vi "Heater Control.vi"(8 "error in":errorcluster, 11 "HeatFlow Results in":refnum<class "Heat Flow Results.lvclass">) -> (0 "error out":errorcluster, 1 "Ugs Cold":dbl caption="Ugs Cold, V", 2 "Ugs Hot":dbl caption="Ugs Hot, V", 3 "HeatFlow Results out":refnum<class "Heat Flow Results.lvclass">)   [LabVIEW 2019, in "Results.lvlib" / "Heat Flow Results.lvclass"]
uses:
  Heat Flow Results.lvclass
  Heat Flow Results.lvclass/Heat Flow Results.ctl
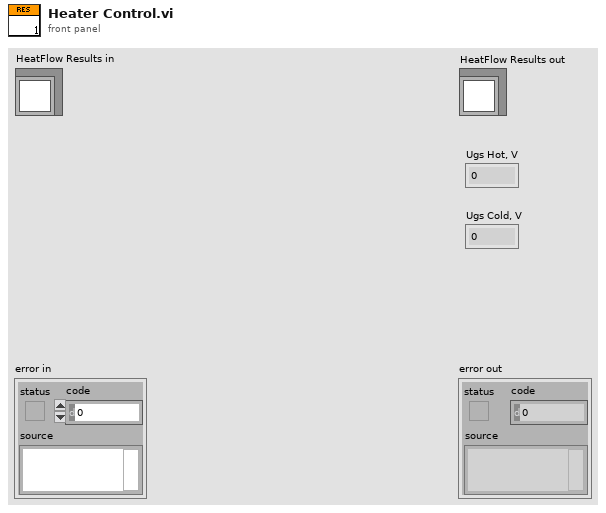
[diagram p1: front panel]
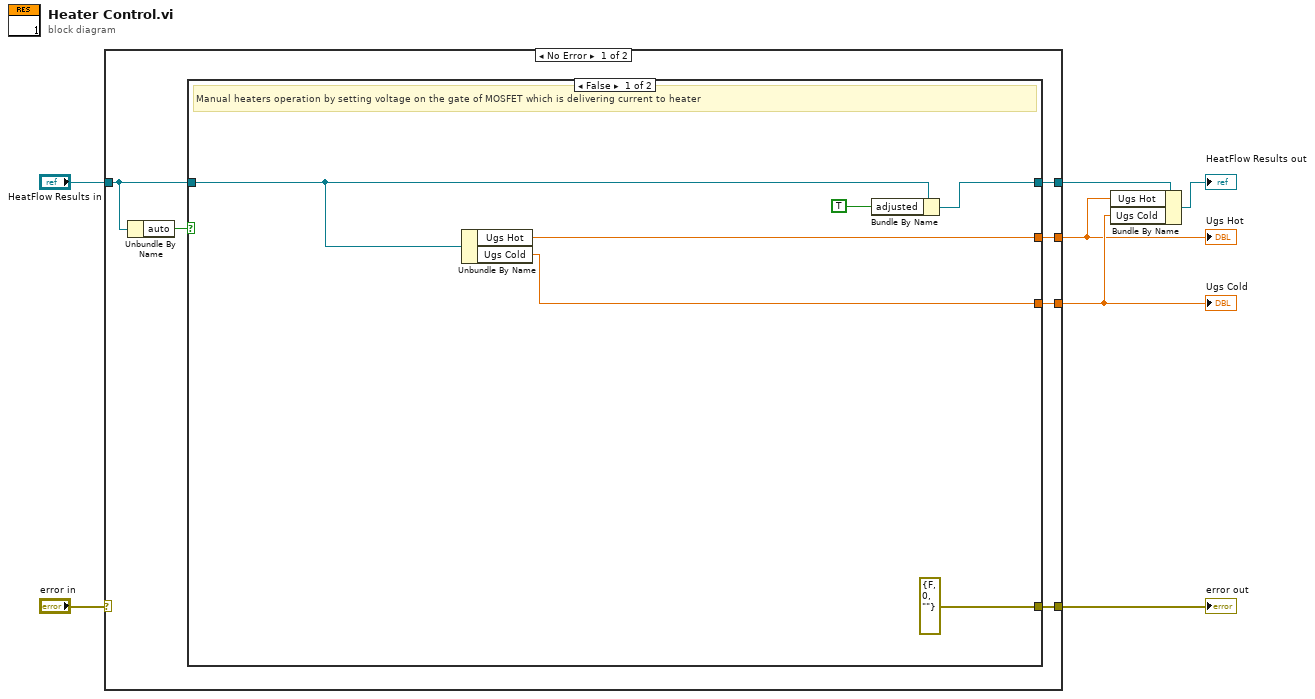
[diagram p0: block diagram]
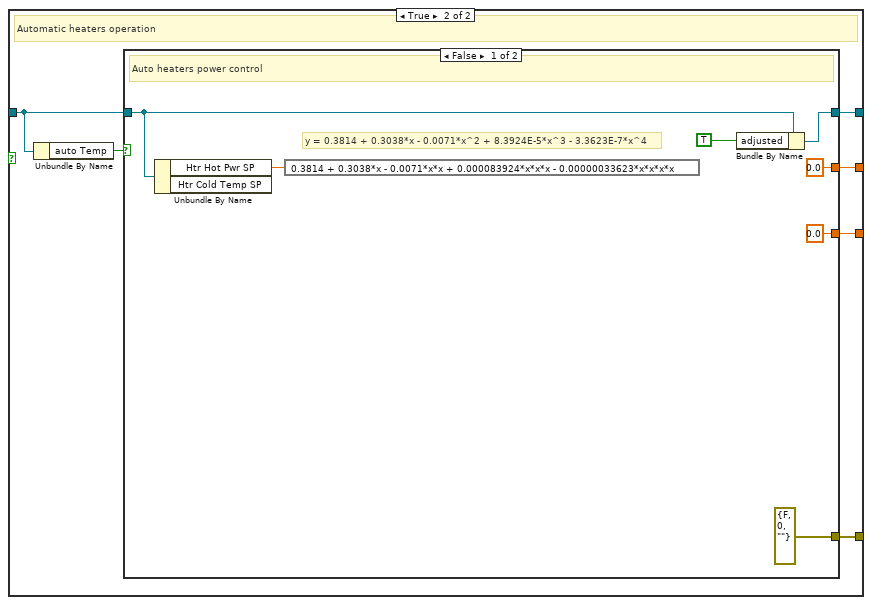
[diagram p2: hidden frame]
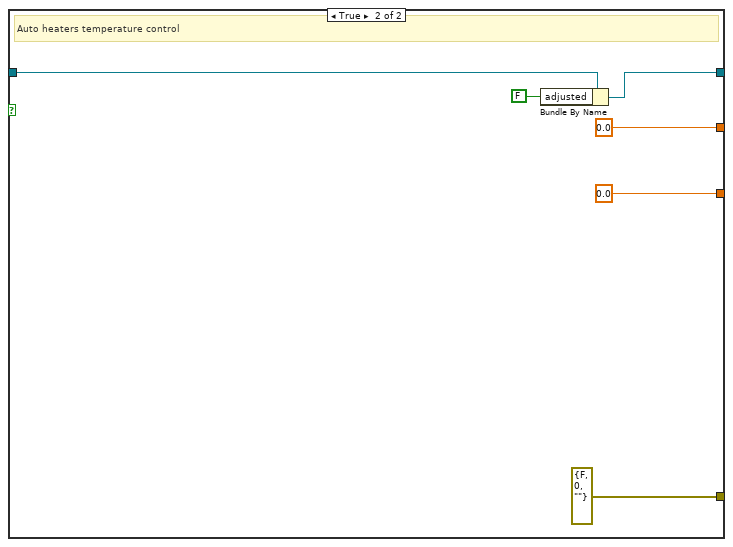
[diagram p3: hidden frame]
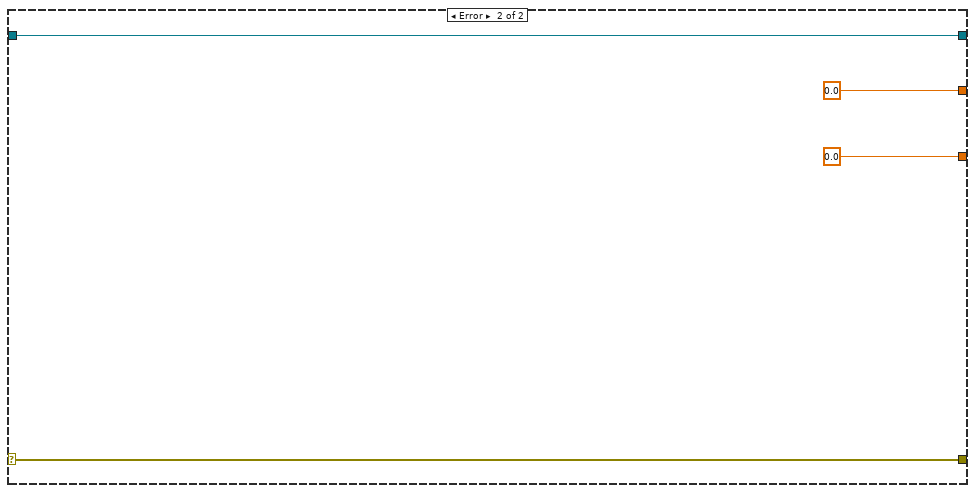
[diagram p4: hidden frame]
diagram:
  n1 = case shown="No Error" "error in" {
    selector: "error in" -> [_ w42]
    tunnel: [w10 w42] -> w6
    tunnel: "HeatFlow Results in" -> [w12 w40]
    tunnel: [w13 0.0 ("Htr MOS Ctrl")] -> w1
    tunnel: [w9 w40] -> w4
    tunnel: [w8 0.0 ("Htr Hot Pwr SP")] -> w2
    frame No Error {
      n2 = Unbundle By Name(w12) -> ("auto"=w11:bool)
      n3 = case shown="False" w11 {
        tunnel: [w19 w23] -> w13
        tunnel: w12 -> [w17 w25]
        tunnel: [errorcluster {"status"=FALSE, "code"=0, "source"=""} ("error IO") w22] -> w10
        tunnel: [w15 w21] -> w9
        tunnel: [w14 w20] -> w8
        frame False {
          # "Manual heaters operation by setting voltage on the gate of MOSFET which is delivering current to heater"
          n4 = Unbundle By Name(w17) -> ("Ugs Hot"=w19:dbl, "Ugs Cold"=w14:dbl)
          n5 = Bundle By Name(cluster=w17, "adjusted"=TRUE) -> (w15:refnum<class "Heat Flow Results.lvclass">)
        }
        frame True {
          # "Automatic heaters operation"
          n6 = Unbundle By Name(w25) -> ("auto Temp"=w24:bool)
          n7 = case shown="False" w24 {
            tunnel: w25 -> [w29 w37]
            tunnel: [0.0 ("Htr Hot Pwr SP") 0.0 ("Htr Hot Pwr SP")] -> w23
            tunnel: [errorcluster {"status"=FALSE, "code"=0, "source"=""} ("error IO") errorcluster {"status"=FALSE, "code"=0, "source"=""} ("error IO")] -> w22
            tunnel: [w31 w36] -> w21
            tunnel: [0.0 ("Htr Hot Pwr SP") 0.0 ("Htr Hot Pwr SP")] -> w20
            frame False {
              # "y = 0.3814 + 0.3038*x - 0.0071*x^2 + 8.3924E-5*x^3 - 3.3623E-7*x^4"
              # "Auto heaters power control"
              n8 = Unbundle By Name(w29) -> ("Htr Hot Pwr SP"=w28:dbl)  [unwired: 1 out]
              n9 = expression code="0.3814 + 0.3038*x - 0.0071*x*x + 0.000083924*x*x*x - 0.00000033623*x*x*x*x"(w28) -> ()  [unwired: 1 out]
              n10 = Bundle By Name(cluster=w29, "adjusted"=TRUE) -> (w31:refnum<class "Heat Flow Results.lvclass">)
            }
            frame True {
              # "Auto heaters temperature control"
              n11 = Bundle By Name(cluster=w37, "adjusted"=FALSE) -> (w36:refnum<class "Heat Flow Results.lvclass">)
            }
          }
        }
      }
    }
    frame Error {
    }
  }
  "error out" <- w6
  "Ugs Hot" <- w1
  "Ugs Cold" <- w2
  n12 = Bundle By Name(cluster=w4, "Ugs Hot"=w1, "Ugs Cold"=w2) -> (→"HeatFlow Results out":refnum<class "Heat Flow Results.lvclass">)
